vi "exchange rate_test_v2.vi"() -> ()   [LabVIEW 2014]
uses:
  <vilib>/Utility/config.llb/Read Key (I32).vi
  <vilib>/Utility/config.llb/Read Key (String).vi
  <vilib>/Utility/config.llb/Write Key (String).vi
  <vilib>/Utility/config.llb/Write Key (I32).vi
  <vilib>/Utility/file.llb/Write To Spreadsheet File (string).vi
  <vilib>/regexp/Match Regular Expression.xnode
  <vilib>/httpClient/LabVIEWHTTPClient.lvlib
  <vilib>/Utility/config.llb/NI_LVConfig.lvlib
panel:
  in  "확인 버튼 2":bool
  out "부분이 삭제된 배열":string[](array[string])
  out "웨이브폼 그래프":i32[](graph)
  out "현재 환율 2":string
  in  "확인 버튼":bool
  in  "world":string(combo)="USD"
  in  "day":string(combo)="13"
  in  "month":string(combo)="08"
  in  "year":string(combo)="2018"
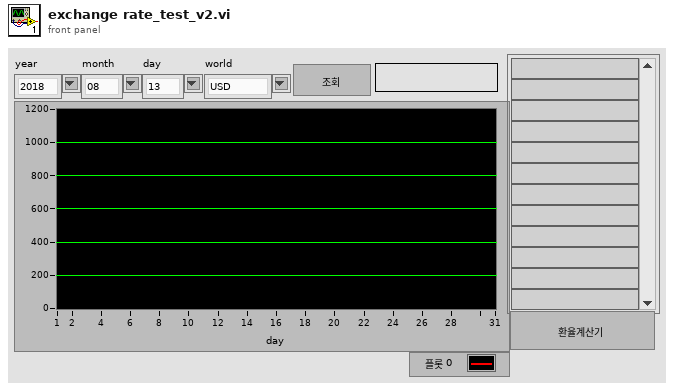
[diagram p1: front panel]
types:
  T1 = typedef "NI_LVConfig.lvlib/Config Data RefNum.ctl" = refnum<k1>
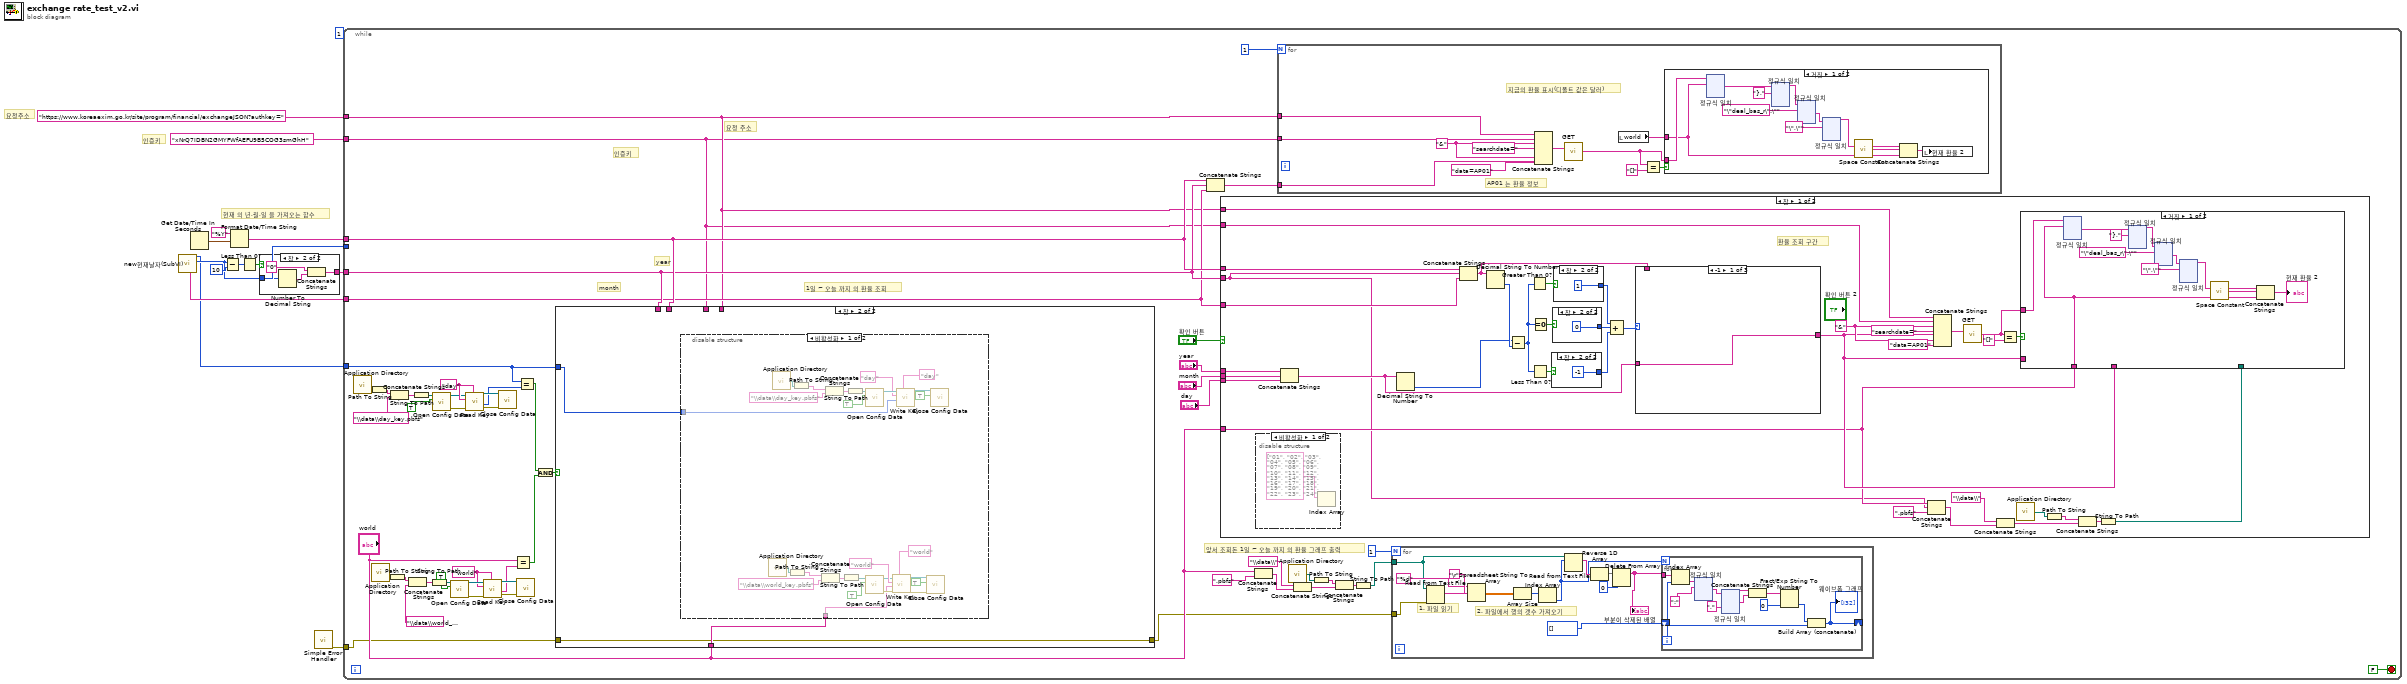
[diagram p0: block diagram]
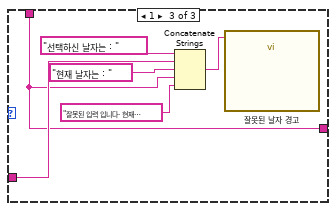
[diagram p5: hidden frame]
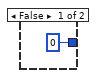
[diagram p6: hidden frame]
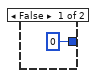
[diagram p7: hidden frame]
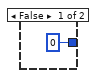
[diagram p8: hidden frame]
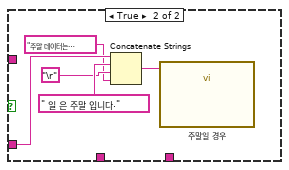
[diagram p9: hidden frame]
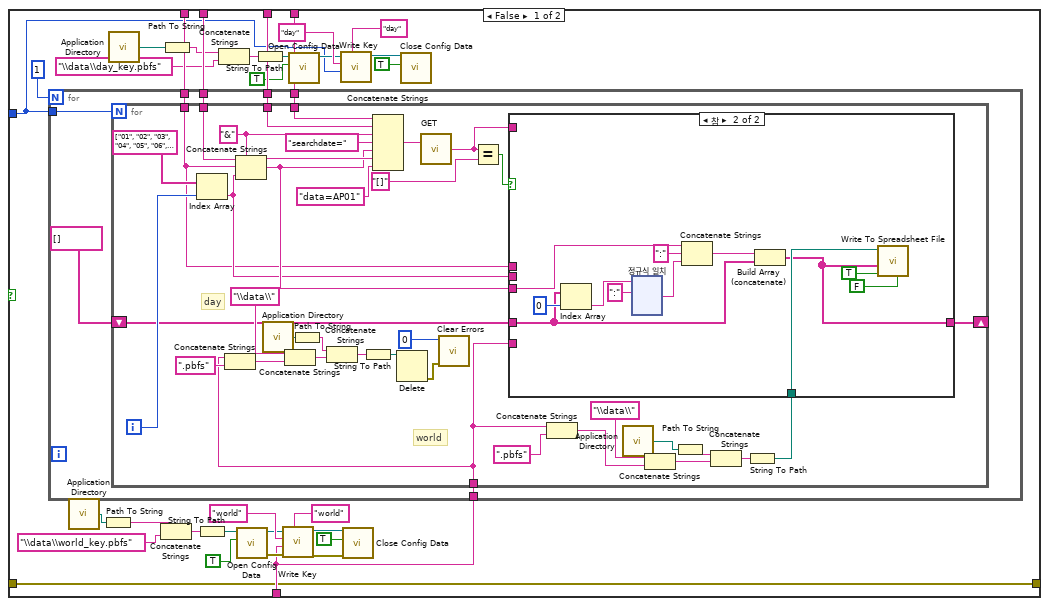
[diagram p11: hidden frame]
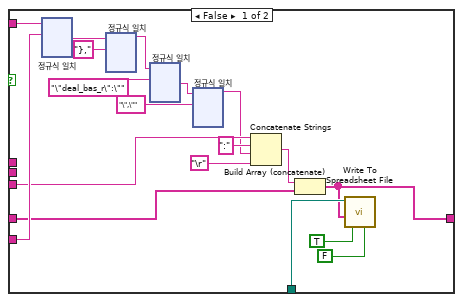
[diagram p12: hidden frame]
diagram:
  (unwired) 1
  # "인증키"
  # "요청주소"
  # "현재 의 년,월,일 을 가져오는 함수"
  n1 = call "new현재날자(SubVI).vi"() -> ("월"=w7:i32, "일"=w3:i32, "일 문자열"=w6:string)  [unwired: 5 in, 4 out]
  n2 = Get Date/Time In Seconds() -> (seconds since 1Jan1904=w10:timestamp)
  n3 = Subtract(x=w7, y=10) -> (x-y=w12:i32)
  n4 = Format Date/Time String(time format string (%c)="%Y" ("시간 포맷 문자열 (%c)"), seconds (now)=w10) -> (date/time string=w8:string)  [unwired: 1 in]
  n5 = Less Than 0?(x=w12) -> (x < 0?=w11:bool)
  n6 = case shown="참" w11 {
    tunnel: w7 -> [_ w17]
    tunnel: [_ w14] -> w2
    frame False {
    }
    frame True {
      n7 = Number To Decimal String(number=w17) -> (decimal integer string=w16:string)  [unwired: 1 in]
      n8 = Concatenate Strings("0", w16) -> (w14:string)
    }
  }
  n9 = call <vilib>:"Simple Error Handler.vi"() -> ("error out"=w1:errorcluster)  [unwired: 5 in, 4 out]
  n10 = while {
    tunnel: w8 -> [w67]
    tunnel: w7 -> [_]
    tunnel: w6 -> [w65]
    tunnel: w2 -> [w66]
    tunnel: "https://www.koreaexim.go.kr/site/program/financial/exchangeJSON?authkey=" -> [w64]
    tunnel: "xNrQ7IDBN2GMYFWfAEFU9B5COG3smGhH" -> [w63]
    tunnel: w3 -> [w69]
    tunnel: w1 -> [w20]
    stop <- FALSE stop-if-true
    w42 = "world" ("key")
    w62 = "day" ("key")
    # "앞서 조회돈 1일 ~ 오늘 까지 의 환율 그래프 출력"
    # "1일 ~ 오늘 까지 의 환율 조회"
    # "year"
    # "month"
    # "요청 주소"
    # "인증키"
    n11 = call <vilib>:"Application Directory.vi"() -> ("Application Directory"=w58:path)
    n12 = Path To String(path=w58) -> (string=w60:string)
    n13 = call <vilib>:"Application Directory.vi"() -> ("Application Directory"=w46:path)
    n14 = Path To String(path=w46) -> (string=w44:string)
    n15 = Concatenate Strings(w60, "\\data\\day_key.pbfs" ("문자열")) -> (w59:string)
    n16 = Concatenate Strings(w44, "\\data\\world_key.pbfs" ("문자열")) -> (w45:string)
    n17 = String To Path(string=w59) -> (path=w61:path)
    n18 = String To Path(string=w45) -> (path=w43:path)
    n19 = call <vilib>:"Open Config Data.vi"("create file if necessary (T)"=TRUE, "configuration file path"=w61) -> ("error out"=w54:errorcluster, "refnum"=w53:T1)  [unwired: 7 in, 1 out]
    n20 = call <vilib>:"Open Config Data.vi"("create file if necessary (T)"=TRUE, "configuration file path"=w43) -> ("error out"=w50:errorcluster, "refnum"=w51:T1)  [unwired: 7 in, 1 out]
    n21 = call-poly <vilib>:"Read Key.vi"("section"=w62, "error in (no error)"=w54, "key"=w62, "refnum"=w53) -> ("error out"=w55:errorcluster, "value"=w52:i32, "refnum out"=w56:T1)  [unwired: 4 in, 1 out]
    n22 = call-poly <vilib>:"Read Key.vi"("section"=w42, "error in (no error)"=w50, "key"=w42, "refnum"=w51) -> ("error out"=w49:errorcluster, "value"=w41:string, "refnum out"=w48:T1)  [unwired: 4 in, 1 out]
    n23 = call <vilib>:"Close Config Data.vi"("error in (no error)"=w55, "refnum"=w56) -> ()  [unwired: 8 in, 2 out]
    n24 = Equal?(x="world", y=w41) -> (x = y?=w39:bool)
    n25 = call <vilib>:"Close Config Data.vi"("error in (no error)"=w49, "refnum"=w48) -> ()  [unwired: 8 in, 2 out]
    n26 = Equal?(x=w69, y=w52) -> (x = y?=w40:bool)
    n27 = And(x=w40, y=w39) -> (x .and. y?=w38:bool)
    n28 = case shown="참" w38 {
      tunnel: w69 -> [w1341 w2002]
      tunnel: w67 -> [w1357 _]
      tunnel: w64 -> [w1356 _]
      tunnel: w63 -> [w1355 _]
      tunnel: w66 -> [w1354 _]
      tunnel: "world" -> [w1327 w2003]
      tunnel: w20 -> [w1326 w2001]
      tunnel: [w1326 w2001] -> w19
      frame False {
        n29 = for {
          N: 1 -> [_]
          tunnel: w1341 -> [w1364]
          tunnel: w1357 -> [w1363]
          tunnel: w1356 -> [w1362]
          tunnel: w1355 -> [w1361]
          tunnel: w1354 -> [w1360]
          tunnel: w1327 -> [w1359]
          n30 = for {
            N: w1364 -> [_]
            tunnel: w1363 -> [w1395]
            tunnel: w1362 -> [w1397]
            tunnel: w1361 -> [w1396]
            tunnel: w1360 -> [w1380]
            tunnel: w1359 -> [w1367]
            shift-right: [w1365] -> _
            shift-left: string[] [] -> [w1366]
            i -> [w1394]
            w1399 = "&" ("문자열")
            # "day"
            # "world"
            n31 = Index Array(array=string[] ["01", "02", "03", "04", "05", "06", "07", "08", "09", "10", "11", "12", "13", "14", "15", "16", "17", "18", "19", "20", "21", "22", "23", "24", "25", "26", "27", "28", "29", "30", "31"], index=w1394) -> (element=w1387:string)
            n32 = Concatenate Strings(w1367, ".pbfs" ("문자열")) -> (w1370:string)
            n33 = Concatenate Strings(w1395, w1380, w1387) -> (w1389:string)
            n34 = call <vilib>:"Application Directory.vi"() -> ("Application Directory"=w1372:path)
            n35 = Concatenate Strings("\\data\\" ("문자열"), w1370) -> (w1369:string)
            n36 = Path To String(path=w1372) -> (string=w1374:string)
            n37 = Concatenate Strings(w1374, w1369) -> (w1373:string)
            n38 = String To Path(string=w1373) -> (path=w1375:path)
            n39 = Concatenate Strings(w1397, w1396, w1399, "searchdate=" ("문자열"), w1389, w1399, "data=AP01" ("문자열")) -> (w1392:string)
            n40 = Delete(path (use dialog)=w1375) -> (error out=w1377:errorcluster)  [unwired: 4 in, 2 out]
            n41 = call <vilib>:"GET.vi"("url"=w1392) -> ("body"=w1390:string)  [unwired: 11 in, 3 out]
            n42 = call <vilib>:"Clear Errors.vi"("error in (no error)"=w1377, "specific error code to clear (0: all)"=0) -> ()  [unwired: 4 in, 2 out]
            n43 = Equal?(x=w1390, y="[]") -> (x = y?=w1391:bool)
            n44 = Concatenate Strings(w1367, ".pbfs" ("문자열")) -> (w1382:string)
            n45 = call <vilib>:"Application Directory.vi"() -> ("Application Directory"=w1384:path)
            n46 = Concatenate Strings("\\data\\" ("문자열"), w1382) -> (w1381:string)
            n47 = Path To String(path=w1384) -> (string=w1386:string)
            n48 = Concatenate Strings(w1386, w1381) -> (w1385:string)
            n49 = String To Path(string=w1385) -> (path=w1379:path)
            n50 = case shown="참" w1391 {
              tunnel: w1389 -> [w1410 w1886]
              tunnel: w1390 -> [w1412 _]
              tunnel: w1367 -> [w1411 _]
              tunnel: w1380 -> [_ _]
              tunnel: w1387 -> [_ _]
              tunnel: w1379 -> [w1407 w1885]
              tunnel: w1366 -> [w1404 w1878]
              tunnel: [w1402 w1879] -> w1365
              frame False {
                n51 = xnode ("정규식 일치")("입력 문자열"=w1412, "정규식"=w1411) -> ("일치 구문 뒤"=w1413:string)  [unwired: 4 in, 4 out]
                n52 = xnode ("정규식 일치")("입력 문자열"=w1413, "정규식"="},") -> ("일치 구문 앞"=w1415:string)  [unwired: 4 in, 4 out]
                n53 = xnode ("정규식 일치")("입력 문자열"=w1415, "정규식"="\"deal_bas_r\":\"") -> ("일치 구문 뒤"=w1417:string)  [unwired: 4 in, 4 out]
                n54 = xnode ("정규식 일치")("입력 문자열"=w1417, "정규식"="\",\"") -> ("일치 구문 앞"=w1408:string)  [unwired: 4 in, 4 out]
                n55 = Concatenate Strings(w1410, ":" ("문자열"), w1408, "\r") -> (w1403:string)
                n56 = Build Array (concatenate)(w1403, w1404) -> (w1402:string[])
                n57 = call-poly <vilib>:"Write To Spreadsheet File.vi"("transpose? (no:F)"=FALSE, "append to file? (new file:F)"=TRUE, "1D data"=w1402, "file path (dialog if empty)"=w1407) -> ()  [unwired: 4 in, 1 out]
              }
              frame True {
                n58 = Index Array(array=w1878, index=0 ("인덱스")) -> (element=w1877:string)
                n59 = xnode "정규식 일치"("입력 문자열"=w1877, "정규식"=":") -> ("일치 구문 뒤"=w1875:string)  [unwired: 4 in, 4 out]
                n60 = Concatenate Strings(w1886, ":", w1875) -> (w1881:string)
                n61 = Build Array (concatenate)(w1881, w1878) -> (w1879:string[])
                n62 = call-poly <vilib>:"Write To Spreadsheet File.vi"("transpose? (no:F)"=FALSE, "append to file? (new file:F)"=TRUE, "1D data"=w1879, "file path (dialog if empty)"=w1885) -> ()  [unwired: 4 in, 1 out]
              }
            }
          }
        }
        n63 = call <vilib>:"Application Directory.vi"() -> ("Application Directory"=w1337:path)
        n64 = Path To String(path=w1337) -> (string=w1339:string)
        n65 = call <vilib>:"Application Directory.vi"() -> ("Application Directory"=w1348:path)
        n66 = Concatenate Strings(w1339, "\\data\\world_key.pbfs" ("문자열")) -> (w1338:string)
        n67 = Path To String(path=w1348) -> (string=w1350:string)
        n68 = String To Path(string=w1338) -> (path=w1340:path)
        n69 = Concatenate Strings(w1350, "\\data\\day_key.pbfs" ("문자열")) -> (w1349:string)
        n70 = call <vilib>:"Open Config Data.vi"("create file if necessary (T)"=TRUE, "configuration file path"=w1340) -> ("error out"=w1329:errorcluster, "refnum"=w1330:T1)  [unwired: 7 in, 1 out]
        n71 = String To Path(string=w1349) -> (path=w1351:path)
        n72 = call-poly <vilib>:"Write Key.vi"("section"="world", "error in (no error)"=w1329, "value"=w1327, "key"="world", "refnum"=w1330) -> ("error out"=w1332:errorcluster, "refnum out"=w1331:T1)  [unwired: 4 in, 1 out]
        n73 = call <vilib>:"Open Config Data.vi"("create file if necessary (T)"=TRUE, "configuration file path"=w1351) -> ("refnum"=w1342:T1)  [unwired: 7 in, 2 out]
        n74 = call-poly <vilib>:"Write Key.vi"("section"="day", "value"=w1341, "key"="day", "refnum"=w1342) -> ("refnum out"=w1343:T1)  [unwired: 5 in, 2 out]
        n75 = call <vilib>:"Close Config Data.vi"("error in (no error)"=w1332, "write file if changed (T)"=TRUE, "refnum"=w1331) -> ()  [unwired: 7 in, 2 out]
        n76 = call <vilib>:"Close Config Data.vi"("write file if changed (T)"=TRUE, "refnum"=w1343) -> ()  [unwired: 8 in, 2 out]
      }
      frame True {
        n77 = disable-structure shown="비활성화" {
          disable-tunnel: w2003 -> [w2005 _]
          disable-tunnel: w2002 -> [w2004 _]
          frame Disabled {
            n78 = call <vilib>:"Application Directory.vi"() -> ("Application Directory"=w2026:path)
            n79 = call <vilib>:"Application Directory.vi"() -> ("Application Directory"=w2011:path)
            n80 = Path To String(path=w2026) -> (string=w2028:string)
            n81 = Path To String(path=w2011) -> (string=w2009:string)
            n82 = Concatenate Strings(w2028, "\\data\\world_key.pbfs" ("문자열")) -> (w2027:string)
            n83 = Concatenate Strings(w2009, "\\data\\day_key.pbfs" ("문자열")) -> (w2010:string)
            n84 = String To Path(string=w2027) -> (path=w2029:path)
            n85 = String To Path(string=w2010) -> (path=w2008:path)
            n86 = call <vilib>:"Open Config Data.vi"("create file if necessary (T)"=TRUE, "configuration file path"=w2029) -> ("error out"=w2018:errorcluster, "refnum"=w2019:T1)  [unwired: 7 in, 1 out]
            n87 = call <vilib>:"Open Config Data.vi"("create file if necessary (T)"=TRUE, "configuration file path"=w2008) -> ("refnum"=w2017:T1)  [unwired: 7 in, 2 out]
            n88 = call-poly <vilib>:"Write Key.vi"("section"="world", "error in (no error)"=w2018, "value"=w2005, "key"="world", "refnum"=w2019) -> ("error out"=w2021:errorcluster, "refnum out"=w2020:T1)  [unwired: 4 in, 1 out]
            n89 = call-poly <vilib>:"Write Key.vi"("section"="day", "value"=w2004, "key"="day", "refnum"=w2017) -> ("refnum out"=w2016:T1)  [unwired: 5 in, 2 out]
            n90 = call <vilib>:"Close Config Data.vi"("error in (no error)"=w2021, "write file if changed (T)"=TRUE, "refnum"=w2020) -> ()  [unwired: 7 in, 2 out]
            n91 = call <vilib>:"Close Config Data.vi"("write file if changed (T)"=TRUE, "refnum"=w2016) -> ()  [unwired: 8 in, 2 out]
          }
          frame Enabled {
          }
        }
      }
    }
    n92 = Concatenate Strings(w67, w66, w65) -> (w22:string)
    n93 = case shown="참" "확인 버튼" {
      tunnel: "world" -> [w811 _]
      tunnel: w65 -> [w810 _]
      tunnel: w67 -> [w809 _]
      tunnel: w66 -> [w802 _]
      tunnel: "month" -> [w806 _]
      tunnel: "day" -> [w807 _]
      tunnel: "year" -> [w805 _]
      tunnel: w64 -> [w804 _]
      tunnel: w63 -> [w803 _]
      frame True {
        w837 = "&" ("문자열")
        # "환율 조회 구간"
        n94 = disable-structure shown="비활성화" {
          frame Disabled {
            n95 = Index Array(array=string[] ["01", "02", "03", "04", "05", "06", "07", "08", "09", "10", "11", "12", "13", "14", "15", "16", "17", "18", "19", "20", "21", "22", "23", "24", "25", "26", "27", "28", "29", "30", "31"]) -> ()  [unwired: 1 in, 1 out]
          }
          frame Enabled {
          }
        }
        n96 = Concatenate Strings(w805, w806, w807) -> (w808:string)
        n97 = Decimal String To Number(string=w808) -> (number=w830:i32)  [unwired: 2 in, 1 out]
        n98 = Concatenate Strings(w809, w802, w810) -> (w821:string)
        n99 = Decimal String To Number(string=w821) -> (number=w831:i32)  [unwired: 2 in, 1 out]
        n100 = Subtract(x=w830, y=w831) -> (x-y=w826:i32)
        n101 = Greater Than 0?(x=w826) -> (x > 0?=w827:bool)
        n102 = Less Than 0?(x=w826) -> (x < 0?=w829:bool)
        n103 = Equal To 0?(x=w826) -> (x = 0?=w828:bool)
        n104 = case shown="참" w829 {
          tunnel: [0 -1] -> w823
          frame False {
          }
          frame True {
          }
        }
        n105 = case shown="참" w828 {
          tunnel: [0 0] -> w824
          frame False {
          }
          frame True {
          }
        }
        n106 = case shown="참" w827 {
          tunnel: [0 1] -> w825
          frame False {
          }
          frame True {
          }
        }
        n107 = Compound Arithmetic op=ADD(w825, w824, w823) -> (w822:i32)
        n108 = case shown="-1" w822 {
          tunnel: w808 -> [w840 _ w846]
          tunnel: w821 -> [_ w841 w844]
          tunnel: [w840 w841 w844] -> w813
          frame -1 {
          }
          frame 0, Default {
          }
          frame 1 {
            n109 = Concatenate Strings("선택하신 날자는 : " ("문자열"), w846, "현재 날자는 : ", w844, "잘못된 입력 입니다. 현재 날자로 검색을 진행 합니다." ("문자열")) -> (w842:string)
            n110 = call "잘못된 날자 경고"("Message"=w842) -> ()  [unwired: 9 in, 2 out]
          }
        }
        n111 = Concatenate Strings(w811, w802, ".pbfs" ("문자열")) -> (w815:string)
        n112 = Concatenate Strings(w804, w803, w837, "searchdate=" ("문자열"), w813, w837, "data=AP01" ("문자열")) -> (w835:string)
        n113 = call <vilib>:"GET.vi"("url"=w835) -> ("body"=w832:string)  [unwired: 11 in, 3 out]
        n114 = Concatenate Strings("\\data\\" ("문자열"), w815) -> (w814:string)
        n115 = Equal?(x=w832, y="[]") -> (x = y?=w833:bool)
        n116 = call <vilib>:"Application Directory.vi"() -> ("Application Directory"=w818:path)
        n117 = Path To String(path=w818) -> (string=w820:string)
        n118 = Concatenate Strings(w820, w814) -> (w819:string)
        n119 = String To Path(string=w819) -> (path=w812:path)
        n120 = case shown="거짓" w833 {
          tunnel: w813 -> [_ w1325]
          tunnel: w832 -> [w856 _]
          tunnel: w811 -> [w855 _]
          tunnel: w813 -> [_ _]
          tunnel: w812 -> [_ _]
          frame False {
            n121 = xnode ("정규식 일치")("입력 문자열"=w856, "정규식"=w855) -> ("일치 구문 뒤"=w857:string)  [unwired: 4 in, 4 out]
            n122 = xnode ("정규식 일치")("입력 문자열"=w857, "정규식"="},") -> ("일치 구문 앞"=w859:string)  [unwired: 4 in, 4 out]
            n123 = xnode ("정규식 일치")("입력 문자열"=w859, "정규식"="\"deal_bas_r\":\"") -> ("일치 구문 뒤"=w861:string)  [unwired: 4 in, 4 out]
            n124 = xnode ("정규식 일치")("입력 문자열"=w861, "정규식"="\",\"") -> ("일치 구문 앞"=w854:string)  [unwired: 4 in, 4 out]
            n125 = call <vilib>:"Space Constant.vi"() -> ("String"=w863:string)
            n126 = Concatenate Strings(w854, w863, w855) -> (→"현재 환율 2":string)
          }
          frame True {
            n127 = Concatenate Strings(w1325, " 일 은 주말 입니다.", "\r", "주말 데이터는 제공되지 않습니다.") -> (w1321:string)
            n128 = call "주말일 경우"("Message"=w1321) -> ()  [unwired: 9 in, 2 out]
          }
        }
      }
      frame False {
      }
    }
    n129 = Concatenate Strings("world", ".pbfs" ("문자열")) -> (w29:string)
    n130 = for {
      N: 1 -> [_]
      tunnel: w22 -> [w330]
      tunnel: w64 -> [w325]
      tunnel: w63 -> [w324]
      w332 = "&" ("문자열")
      # "지금의 환율 표시(디폴트 값은 달러)"
      # "AP01 는 환율 정보"
      n131 = Concatenate Strings(w325, w324, w332, "searchdate=" ("문자열"), w330, w332, "data=AP01" ("문자열")) -> (w334:string)
      n132 = call <vilib>:"GET.vi"("url"=w334) -> ("body"=w326:string)  [unwired: 11 in, 3 out]
      n133 = local read "world"() -> (w329:string)
      n134 = Equal?(x=w326, y="[]") -> (x = y?=w327:bool)
      n135 = case shown="거짓" w327 {
        tunnel: w326 -> [w338 _]
        tunnel: w329 -> [w336 _]
        frame False {
          n136 = xnode ("정규식 일치")("입력 문자열"=w338, "정규식"=w336) -> ("일치 구문 뒤"=w339:string)  [unwired: 4 in, 4 out]
          n137 = xnode ("정규식 일치")("입력 문자열"=w339, "정규식"="},") -> ("일치 구문 앞"=w341:string)  [unwired: 4 in, 4 out]
          n138 = xnode ("정규식 일치")("입력 문자열"=w341, "정규식"="\"deal_bas_r\":\"") -> ("일치 구문 뒤"=w343:string)  [unwired: 4 in, 4 out]
          n139 = xnode ("정규식 일치")("입력 문자열"=w343, "정규식"="\",\"") -> ("일치 구문 앞"=w337:string)  [unwired: 4 in, 4 out]
          n140 = call <vilib>:"Space Constant.vi"() -> ("String"=w345:string)
          n141 = Concatenate Strings(w337, w345, w336) -> (w335:string)
          n142 = local write "현재 환율 2"(w335) -> ()
        }
        frame True {
        }
      }
    }
    n143 = call <vilib>:"Application Directory.vi"() -> ("Application Directory"=w32:path)
    n144 = Concatenate Strings("\\data\\" ("문자열"), w29) -> (w28:string)
    n145 = Path To String(path=w32) -> (string=w34:string)
    n146 = Concatenate Strings(w34, w28) -> (w33:string)
    n147 = String To Path(string=w33) -> (path=w35:path)
    n148 = for {
      N: 1 -> [_]
      tunnel: w35 -> [w77]
      tunnel: w19 -> [w70]
      # "2. 파일에서 행의 갯수 가져오기"
      # "1. 파일 읽기"
      n149 = Read from Text File(file (use dialog)=w77, error in=w70) -> (text=w82:string)  [unwired: 5 out]
      n150 = Spreadsheet String To Array(delimiter (Tab)="\r", format string="%d", spreadsheet string=w82) -> (array=w80:dbl[][])  [unwired: 1 out]
      n151 = Array Size(array=w80) -> (size(s)=w81:i32[])
      n152 = Index Array(array=w81) -> (element=w74:i32)  [unwired: 1 in]
      n153 = Read from Text File(file (use dialog)=w77, count=w74) -> (text=w75:string[])  [unwired: 1 in, 4 out]
      n154 = Reverse 1D Array(array=w75) -> (reversed array=w73:string[])
      n155 = Delete From Array(array=w73, index=0 ("인덱스")) -> (array with subset deleted=w72:string[])  [unwired: 1 in, 1 out]
      "부분이 삭제된 배열" <- w72
      n156 = for {
        N: w74 -> [_]
        tunnel: w72 -> [w89]
        shift-right: [w87] -> _
        shift-left: i32[] [] -> [w88]
        i -> [w90]
        n157 = Index Array(array=w89, index=w90) -> (element=w95:string)
        n158 = xnode "정규식 일치"("입력 문자열"=w95, "정규식"=":") -> ("일치 구문 뒤"=w86:string)  [unwired: 4 in, 4 out]
        n159 = xnode "정규식 일치"("입력 문자열"=w86, "정규식"=",") -> ("일치 구문 앞"=w92:string, "일치 구문 뒤"=w91:string)  [unwired: 4 in, 3 out]
        n160 = Concatenate Strings(w92, w91) -> (w85:string)
        n161 = Fract/Exp String To Number(string=w85, default (0 dbl)=0) -> (number=w84:i32)  [unwired: 2 in, 1 out]
        n162 = Build Array (concatenate)(w84, w88) -> (w87:i32[])
        "웨이브폼 그래프" <- w87
      }
    }
  }
